vi "GyroDirve.vi"(0 "NXT":T1, 1 "Left Drive":cluster{T2, T2}, 3 "Right Drive":cluster{T2, T2}, 4 "Port/MUX":T3 {"Port" items=["Port 1", "Port 2", "Port 3", "Port 4"]; "MUX Port" items=["No MUX", "MUX 1", "MUX 2", "MUX 3", "MUX 4"]}) -> (7 "NXT 2":T1)   [LabVIEW 2012]
uses:
  <vilib>/NXT/LegoClasses/BrickReference/BrickReference.lvclass
  <vilib>/NXT/Subs/LVHSConnector.ctl
  <vilib>/NXT/NXTIO Xnodes/NXTIOXNode/NXTIO.xnode
  <vilib>/NXT/Hardware/Plugins/Open Port/OpenPortAddress.ctl
  <vilib>/NXT/Block Support/NXT_InputPort.ctl
  <vilib>/NXT/HiTechnic/HiTechnic Controls/HiTechnic Port.ctl
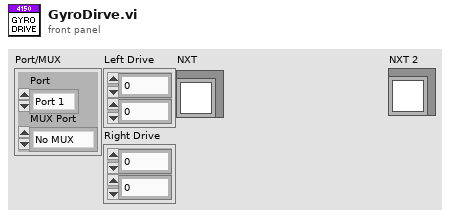
[diagram p1: front panel]
types:
  T1 = typedef "LVHSConnector.ctl" = refnum<class "BrickReference.lvclass">
  T2 = typedef "OpenPortAddress.ctl" = i32
  T3 = typedef "HiTechnic Port.ctl" = cluster{"Port":T4, "MUX Port":u8}
  T4 = typedef "NXT_InputPort.ctl" = u8
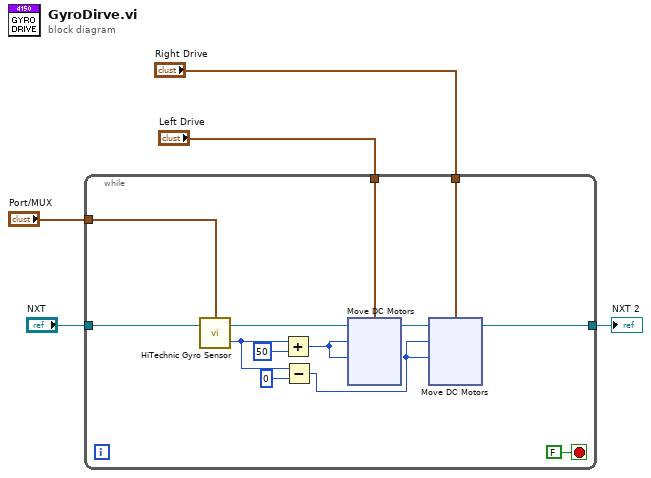
[diagram p0: block diagram]
diagram:
  n1 = while {
    tunnel: "Left Drive" -> [w17]
    tunnel: "Port/MUX" -> [w16]
    tunnel: "Right Drive" -> [w14]
    tunnel: "NXT" -> [w7]
    tunnel: [w6] -> w1
    stop <- FALSE stop-if-true
    n2 = call <vilib>:"HiTechnic Gyro Sensor.vi"("NXT"=w7, "Port/MUX"=w16) -> ("Gyro Value"=w10:i16, "NXT"=w13:T1)  [unwired: 1 in]
    n3 = Add(x=w10, y=i16 50) -> (x+y=w8:i16)
    n4 = Subtract(x=w10, y=i16 0) -> (x-y=w9:i16)
    n5 = xnode "Move DC Motors"("Power/Speed 2"=w8, "Power/Speed 1"=w8, "Motors"=w17, "NXT"=w13) -> ("NXT"=w15:T1)
    n6 = xnode "Move DC Motors"("Power/Speed 2"=w9, "Power/Speed 1"=w9, "Motors"=w14, "NXT"=w15) -> ("NXT"=w6:T1)
  }
  "NXT 2" <- w1
